vi "InitExoskeletonObject.vi"(6 "Loop Period":dbl=0.025) -> (0 "error out":errorcluster, 3 "Exoskeleton Object":refnum<class "Exoskeleon.lvclass">)   [LabVIEW 2014, in "Exoskeleon.lvclass"]
uses:
  Classes/CAREX_Classes_old/Exoskeleton/Exoskeleon.lvclass
  <vilib>/imath/engines/lvmath2/RunTimeEngine/Managers/WorkSpace/UID Generator.vi
  <vilib>/imath/engines/lvmath2/RunTimeEngine/RangeToken/NIMS_Range_R2 - Integer.vi
  <instcachedir>/0/NIMS_Range_R2 - Integer_2D1304BAF97744E0A293025746CBADFC.lvgen/NIMS_Range_R2 - Integer_2D1304BAF97744E0A293025746CBADFC_000.vi
  <vilib>/imath/engines/lvmath2/RunTimeEngine/CommandStatement/MC_CommandStatement_break.vi
  <vilib>/imath/engines/lvmath2/RunTimeEngine/IndexRead/NIMS V(S).vi
  <instcachedir>/0/NIMS V(S)_0488751826AF41519A22953C041130DC.lvgen/NIMS V(S)_0488751826AF41519A22953C041130DC_000.vi
  <vilib>/imath/engines/lvmath2/RunTimeEngine/IndexReplace/NIMS M(R2,S)=V.vi
  <instcachedir>/0/NIMS M(R2,S)=V_7A59E123E5EA412A8382473AE7186B5F.lvgen/NIMS M(R2,S)=V_7A59E123E5EA412A8382473AE7186B5F_000.vi
  <vilib>/imath/engines/lvmath2/RunTimeEngine/ErrorHandling/NIMS_Create Error From Enums.vi
  <vilib>/imath/engines/lvmath2/RunTimeEngine/ArithmeticOperatorToken/NIMS_ArithmeticOperator_plus.vi
  <instcachedir>/0/NIMS_ArithmeticOperator_plus_48D6EAACA5D645B09F7EC9C016C2DEA8.lvgen/NIMS_ArithmeticOperator_plus_48D6EAACA5D645B09F7EC9C016C2DEA8_004.vi
  <vilib>/imath/engines/lvmath2/RunTimeEngine/IndexRead/NIMS M(R2,S).vi
  <instcachedir>/0/NIMS M(R2,S)_56813DCFDD5A484292D2195AF15D2BF5.lvgen/NIMS M(R2,S)_56813DCFDD5A484292D2195AF15D2BF5_000.vi
  <vilib>/imath/engines/lvmath2/RunTimeEngine/RunTimeType/NIMS_RunTimeType_From StrictType (excl LVString).vi
  <instcachedir>/0/NIMS_RunTimeType_From StrictType (excl LVString)_15A5391EEA9C4AACB9955AC755B83D29.lvgen/NIMS_RunTimeType_From StrictType (excl LVString)_15A5391EEA9C4AACB9955AC755B83D29_000.vi
  <vilib>/imathl/engines/lvmath/Functions/Error Handling/Create Error.vi
  <vilib>/imath/engines/lvmath2/RunTimeEngine/LocalVariableDefStatement/MC_LocalVariableDefStatement_Display.vi
  <vilib>/imath/engines/lvmath2/RunTimeEngine/IndexRead/NIMS M(S,S).vi
  <instcachedir>/0/NIMS M(S,S)_AC51E74150A542F7991B9634C66F3096.lvgen/NIMS M(S,S)_AC51E74150A542F7991B9634C66F3096_000.vi
  <vilib>/imath/engines/lvmath2/RunTimeEngine/IndexReplace/NIMS M(S,S)=S.vi
  <instcachedir>/0/NIMS M(S,S)=S_43446D47E75543269C90719353EB0EB0.lvgen/NIMS M(S,S)=S_43446D47E75543269C90719353EB0EB0_000.vi
  <vilib>/imath/engines/lvmath2/RunTimeEngine/Managers/SymbolTable/Clear UID.vi
  <vilib>/imath/engines/lvmath2/RunTimeEngine/NodeEndStatement/NIMS_NodeEndStatement_Output.vi
  <instcachedir>/0/NIMS_NodeEndStatement_Output_53EC0D466D134D7ABD903AC30B43404B.lvgen/NIMS_NodeEndStatement_Output_53EC0D466D134D7ABD903AC30B43404B_002.vi
  <vilib>/imath/engines/lvmath2/RunTimeEngine/ErrorHandling/NIMS_Finalize Error.vi
  Classes/CAREX_Classes_old/Exoskeleton/Exoskeleton_SetLinkMass.vi
  Classes/CAREX_Classes_old/Exoskeleton/Exoskeleton_SetLinkCOMs.vi
  Classes/CAREX_Classes_old/Exoskeleton/Exoskeleton_SetTensionLimits.vi
  Classes/CAREX_Classes_old/Exoskeleton/Exoskeleton_SetLoopPeriod.vi
  Classes/CAREX_Classes_old/Exoskeleton/Exoskeleton_SetCableMapping.vi
  Classes/CAREX_Classes_old/Exoskeleton/Exoskeleton_SetCableAttachmentPts.vi
  <vilib>/imath/engines/lvmath2/RunTimeEngine/Managers/SymbolTable/NIMS_WorkSpace.lvlib
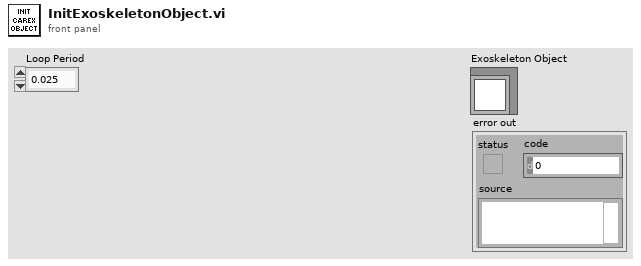
[diagram p1: front panel]
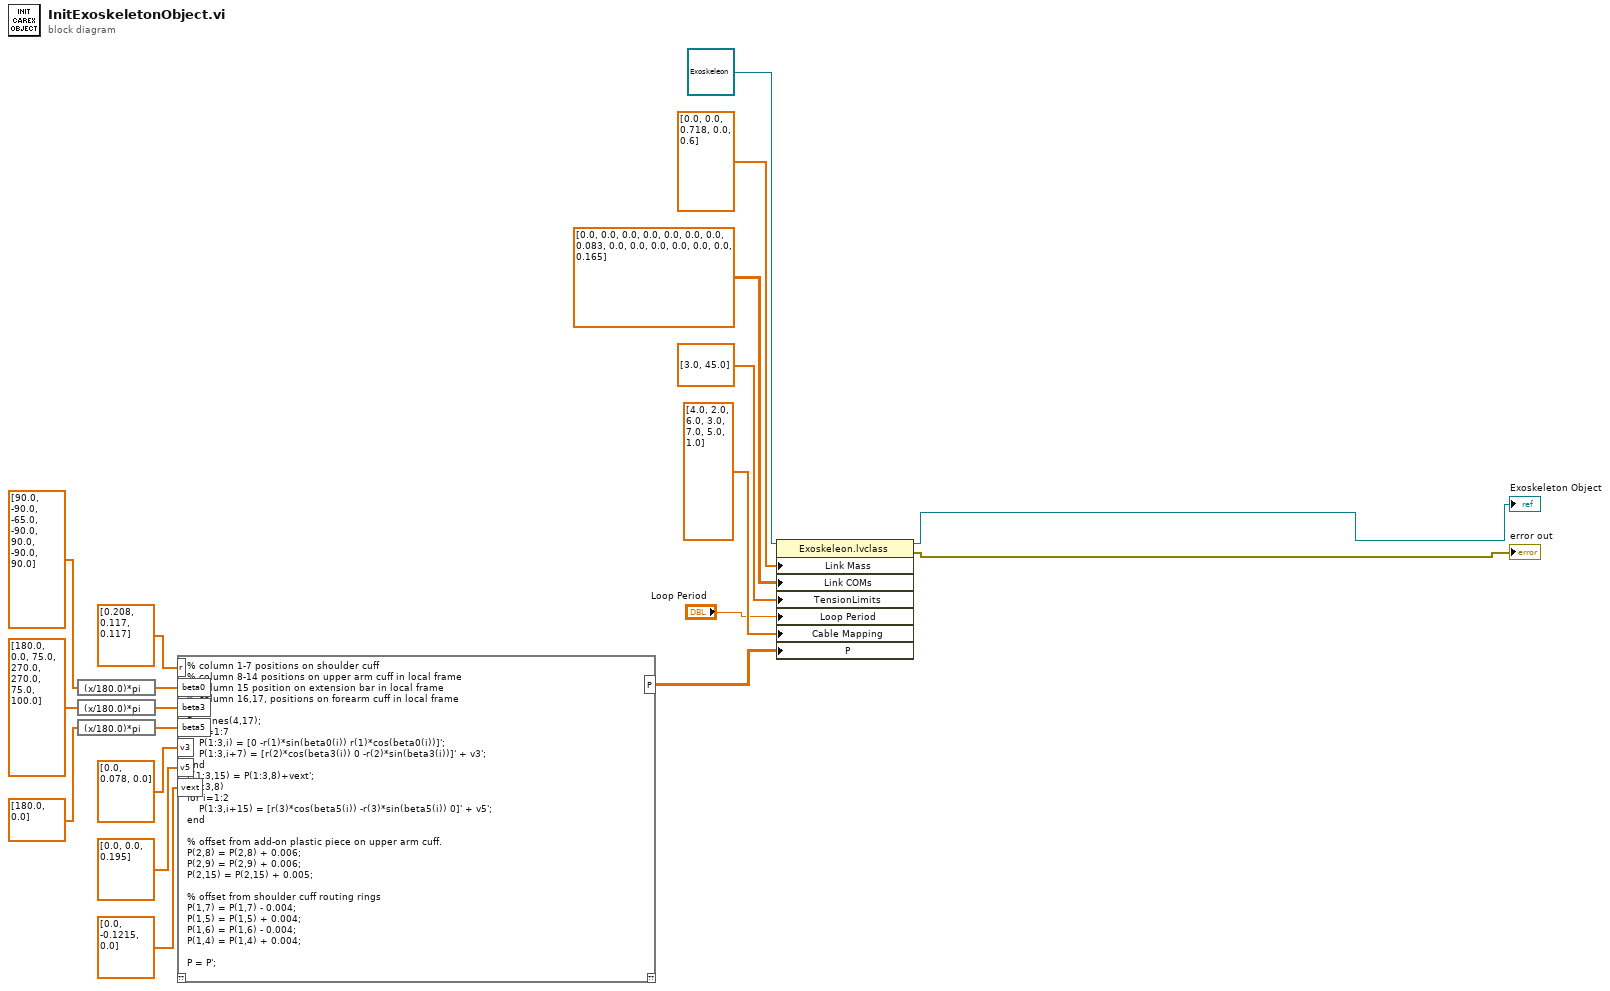
[diagram p0: block diagram]
diagram:
  n1 = expression code="(x/180.0)*pi" ("degrees to radians")(dbl[] [90.0, -90.0, -65.0, -90.0, 90.0, -90.0, 90.0]) -> (w9:dbl[])
  n2 = expression code="(x/180.0)*pi" ("degrees to radians")(dbl[] [180.0, 0.0, 75.0, 270.0, 270.0, 75.0, 100.0]) -> (w8:dbl[])
  n3 = expression code="(x/180.0)*pi" ("degrees to radians")(dbl[] [180.0, 0.0]) -> (w7:dbl[])
  n4 = mathscript code="% column 1-7 positions on shoulder cuff\n% column 8-14 positions on upper arm cuff in local frame\n% column 15 position on extension bar in local frame\n% column 16,17, positions on forearm cuff in local frame\n\nP = ones(4,17);\nfor i=1:7\n    P(1:3,i) = [0 -r(1)*sin(beta0(i)) r(1)*cos(beta0(i))]';\n    P(1:3,i+7) = [r(2)*cos(beta3(i)) 0 -r(2)*sin(beta3(i))]' + v3';\nend\nP(1:3,15) = P(1:3,8)+vext';\nP(1:3,8)\nfor i=1:2\n    P(1:3,i+15) = [r(3)*cos(beta5(i)) -r(3)*sin(beta5(i)) 0]' + v5';\nend\n\n% offset from add-on plastic piece on upper arm cuff.\nP(2,8) = P(2,8) + 0.006;\nP(2,9) = P(2,9) + 0.006;\nP(2,15) = P(2,15) + 0.005;\n\n% offset from shoulder cuff routing rings\nP(1,7) = P(1,7) - 0.004;\nP(1,5) = P(1,5) + 0.004;\nP(1,6) = P(1,6) - 0.004;\nP(1,4) = P(1,4) + 0.004;\n\nP = P';"("r"=dbl[] [0.208, 0.117, 0.117], "beta0"=w9, "beta3"=w8, "beta5"=w7, "v3"=dbl[] [0.0, 0.078, 0.0], "v5"=dbl[] [0.0, 0.0, 0.195], "vext"=dbl[] [0.0, -0.1215, 0.0]) -> ("P"=w3:dbl[][])  [unwired: 1 in, 1 out]
  n5 = property class="Exoskeleon.lvclass"(reference=refnum<class "Exoskeleon.lvclass"> refnum ("Exoskeleon.lvclass"), "Link Mass"=dbl[] [0.0, 0.0, 0.718, 0.0, 0.6], "Link COMs"=dbl[][] [[0.0, 0.0, 0.0], [0.0, 0.0, 0.0], [0.0, 0.083, 0.0], [0.0, 0.0, 0.0], [0.0, 0.0, 0.165]], "TensionLimits"=dbl[] [3.0, 45.0], "Loop Period"="Loop Period", "Cable Mapping"=dbl[] [4.0, 2.0, 6.0, 3.0, 7.0, 5.0, 1.0], "P"=w3) -> (reference out=→"Exoskeleton Object":refnum<class "Exoskeleon.lvclass">, error out=→"error out":errorcluster)  [unwired: 1 in]
